vi "Ejercicio 2.2.vi"() -> ()   [LabVIEW 2020]
uses:
  <vilib>/numeric/sub_Random U32.vi
  <vilib>/numeric/Random Number (Range) U64.vi
panel:
  out "min value":dbl
  out "max value":dbl
  out "Filtro EMA":dbl[](graph)
  out "?":dbl[][](array[numeric])
  out "Valores aleatoreos de la temperatura C°":u64[](graph)
  # "C°"
  # "F°"
  # "EMA"
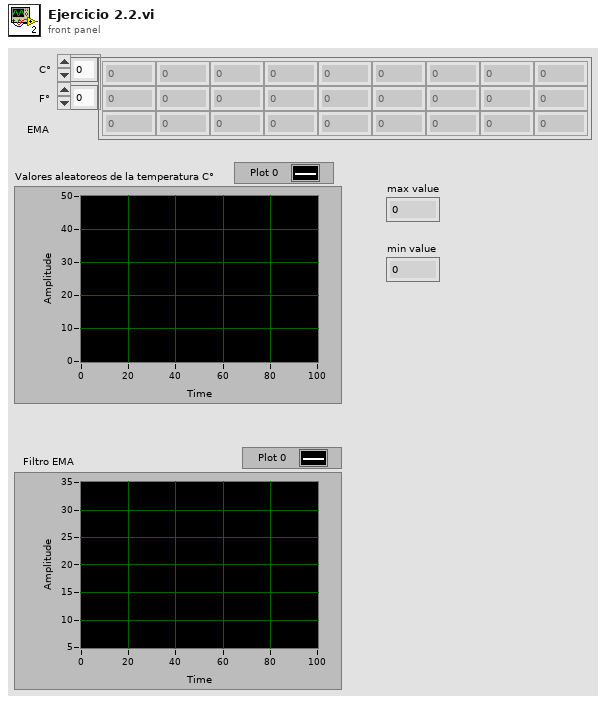
[diagram p1: front panel]
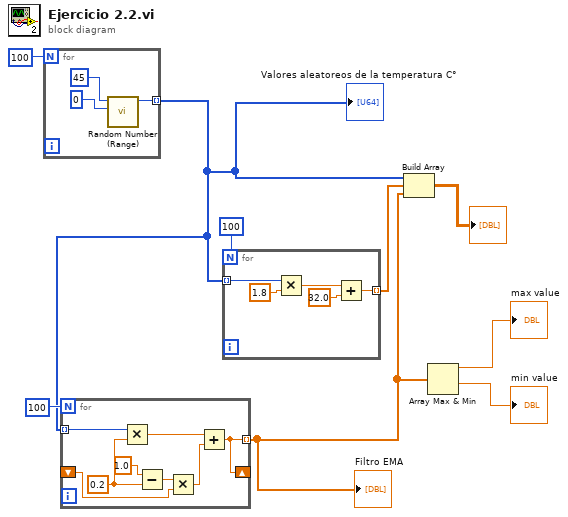
[diagram p0: block diagram]
diagram:
  n1 = for {
    N: 100 -> [_]
    tunnel: [w10] -> w4 mode=indexing
    n2 = call-poly <vilib>:"Random Number (Range).vi"("lower bound (0)"=u64 0, "upper bound (100)"=u64 45) -> ("number"=w10:u64)  [unwired: 9 in]
  }
  "Valores aleatoreos de la temperatura C°" <- w4
  n3 = for {
    N: 100 -> [_]
    shift-right: [w14] -> _
    shift-left: _ -> [w15]
    tunnel: [w14] -> w3 mode=indexing
    tunnel: w4 -> [w13] mode=indexing
    w18 = 0.2 ("y")
    n4 = Multiply(x=w13, y=w18) -> (x*y=w20:dbl)
    n5 = Subtract(x=1.0, y=w18) -> (x-y=w17:dbl)
    n6 = Multiply(x=w17, y=w15) -> (x*y=w16:dbl)
    n7 = Add(x=w20, y=w16) -> (x+y=w14:dbl)
  }
  "Filtro EMA" <- w3
  n8 = for {
    N: 100 -> [_]
    tunnel: w4 -> [w25] mode=indexing
    tunnel: [w21] -> w5 mode=indexing
    n9 = Multiply(x=w25, y=1.8) -> (x*y=w23:dbl)
    n10 = Add(x=w23, y=32.0) -> (x+y=w21:dbl)
  }
  n11 = Build Array(w4, w5, w3) -> (→"?":dbl[][])
  n12 = Array Max & Min(array=w3) -> (max value=→"max value":dbl, min value=→"min value":dbl)  [unwired: 2 out]
